vi "copyFromIniToTable.vi"(0 "Tbl Refnum in":refnum<vi>, 1 "valInCol5":string, 5 "Tree Refnum in":refnum<vi>, 7 "valInCol1":string, 9 "valInCol2":string, 11 "error in":errorcluster, 12 "tableRowNum":u32) -> (4 "Tbl Refnum out":refnum<vi>, 6 "Tree Refnum out":refnum<vi>, 8 "col1FoundInTree?":bool, 15 "error out":errorcluster)   [LabVIEW 2010]
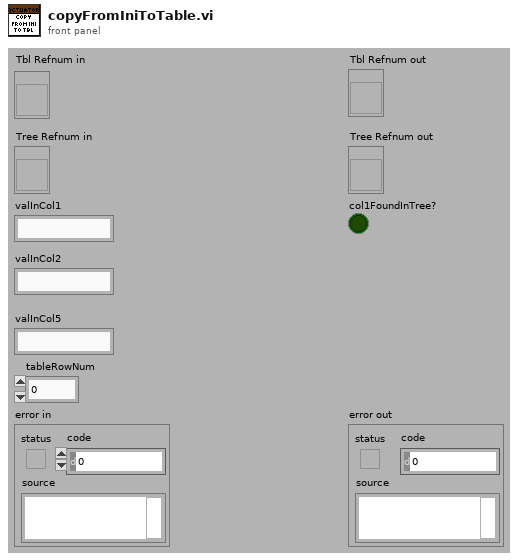
[diagram p1: front panel]
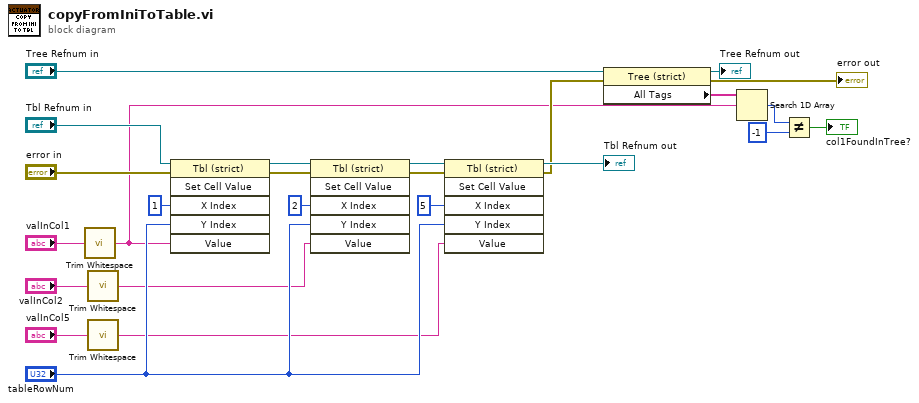
[diagram p0: block diagram]
diagram:
  n1 = call <vilib>:"Trim Whitespace.vi"("string"="valInCol1") -> ("trimmed string"=w6:string)  [unwired: 1 in]
  n2 = call <vilib>:"Trim Whitespace.vi"("string"="valInCol2") -> ("trimmed string"=w9:string)  [unwired: 1 in]
  n3 = call <vilib>:"Trim Whitespace.vi"("string"="valInCol5") -> ("trimmed string"=w7:string)  [unwired: 1 in]
  n4 = invoke class="Tbl (strict)" method="Set Cell Value"(reference="Tbl Refnum in", error in="error in", "X Index"=u32 1, "Y Index"="tableRowNum", "Value"=w6) -> (reference out=w22:refnum<vi>, error out=w23:errorcluster)  [unwired: 1 in, 4 out]
  n5 = invoke class="Tbl (strict)" method="Set Cell Value"(reference=w22, error in=w23, "X Index"=u32 2, "Y Index"="tableRowNum", "Value"=w9) -> (reference out=w21:refnum<vi>, error out=w20:errorcluster)  [unwired: 1 in, 4 out]
  n6 = invoke class="Tbl (strict)" method="Set Cell Value"(reference=w21, error in=w20, "X Index"=u32 5, "Y Index"="tableRowNum", "Value"=w7) -> (reference out=→"Tbl Refnum out":refnum<vi>, error out=w14:errorcluster)  [unwired: 1 in, 4 out]
  n7 = property on="Property Node" class="Tree (strict)"(reference="Tree Refnum in", error in=w14) -> (reference out=→"Tree Refnum out":refnum<vi>, error out=→"error out":errorcluster, "All Tags"=w12:string[])
  n8 = Search 1D Array(1D array=w12, element=w6) -> (index of element=w3:i32)  [unwired: 1 in]
  n9 = Not Equal?(x=w3, y=-1) -> (x != y?=→"col1FoundInTree?":bool)
